vi "Ultrasonico.vi"() -> ()   [LabVIEW 2016]
panel:
  in  "error in (no error)":errorcluster
  out "Value":u16(slide) scale=0.0..250.0
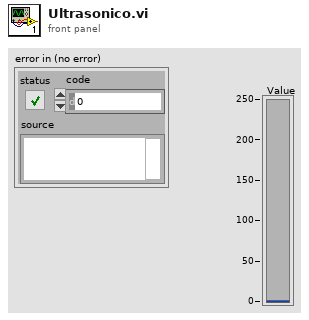
[diagram p1: front panel]
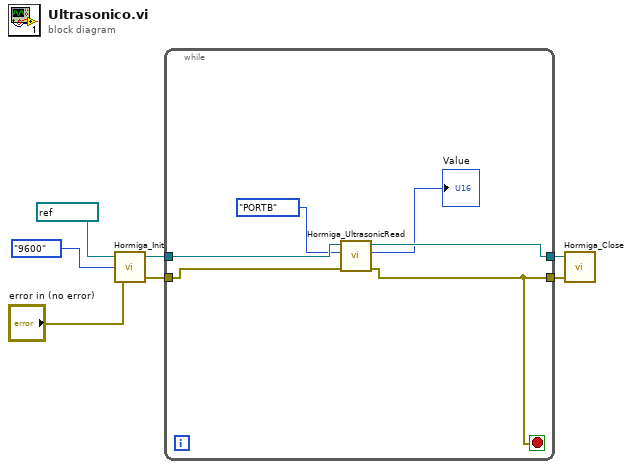
[diagram p0: block diagram]
diagram:
  n1 = call "Hormiga_Init.vi"("error in (no error)"="error in (no error)", "Velocidad de Conexion"=enum16{"115200", "9600"}."9600", "VISA Refnum in"=refnum<visa-resource-name> "COM5") -> ("error out"=w7:errorcluster, "VISA Refnum out"=w6:refnum<visa-resource-name>)  [unwired: 1 in]
  n2 = while {
    tunnel: w7 -> [w13]
    tunnel: w6 -> [w12]
    tunnel: [w8] -> w5
    tunnel: [w11] -> w4
    stop <- w8 stop-if-true
    n3 = call "Hormiga_UltrasonicRead.vi"("error in (no error)"=w13, "Puerto"=enum32{"PORTB", "PORTD"}."PORTB", "VISA Refnum in"=w12) -> ("error out"=w8:errorcluster, "Value"=→"Value":u16, "VISA Refnum out"=w11:refnum<visa-resource-name>)  [unwired: 6 in]
  }
  n4 = call "Hormiga_Close.vi"("error in (no error)"=w5, "VISA Refnum in"=w4) -> ()  [unwired: 2 in]
